vi "getAttribute_action.vi"(0 "HGF_ImaqDx":refnum<class "HGF_ImaqDx.lvclass">, 1 "Attribute Name":string, 5 "error in (no error)":errorcluster) -> (14 "dup HGF_ImaqDx":refnum<class "HGF_ImaqDx.lvclass">, 15 "IMAQdx Attribute":variant, 19 "error out":errorcluster)   [LabVIEW 2014, in "HGF_IMAQ.lvlib" / "HGF_ImaqDx.lvclass"]
doc: "Return the name of camera."
uses:
  HGF_ImaqDx.lvclass
  HGF_IMAQDevice/HGF_IMAQDevice.lvclass
  HGF_Auxiliary/HGF_Auxiliary.lvlib
  HGF_Auxiliary/Severity.ctl
  HGF_Auxiliary/ErrorCode.ctl
  VisionTools/HGF_VisionTools/HGF_VisionTools.lvlib
  VisionTools/HGF_VisionTools/IMAQdx_getAttribute_Bool.vi
  VisionTools/HGF_VisionTools/IMAQdx_getAttribute_I64.vi
  VisionTools/HGF_VisionTools/IMAQdx_getAttribute_Dbl.vi
  VisionTools/HGF_VisionTools/IMAQdx_getAttribute_U32.vi
  VisionTools/HGF_VisionTools/IMAQdx_getAttribute_Str.vi
  VisionTools/HGF_VisionTools/IMAQdx_getAttribute_Enum.vi
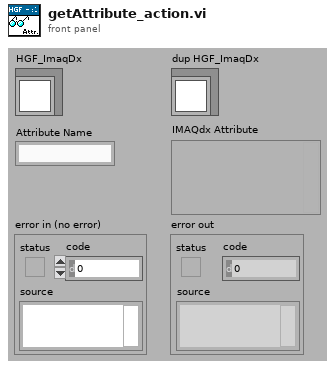
[diagram p1: front panel]
types:
  T1 = typedef "HGF_Auxiliary.lvlib/ErrorCode.ctl" = enum32{"No error", "Function not supported.", "This VI is for friends only.", "Reference object aready exisits.", "Parameter out of range.", "Not a rendezvous.", "Invalid notifier reference.", "Invalid queue reference.", "Self-Test not supported.", "Reset not supported.", "IDN query not supported.", "Error query not supported.", "Incorrect addressee.", "Object already exists.", "No class name specified", "Driver not supported", "Attribute is not writable"}
  T2 = typedef "HGF_Auxiliary.lvlib/Severity.ctl" = enum16{"Info", "Warning", "Fault", "Error", "Fatal"}
  T3 = typedef "NI_Vision_Acquisition_Software.lvlib/IMAQdx Attribute Type.ctl" = enum32{"U32", "I64", "DBL", "String", "Enum", "Bool", "Command"}
  T4 = cluster{"Attribute Type":T3, "Readable":bool, "Writable":bool, "Attribute Name":string}[]
  T5 = cluster{"Attribute Type":T3, "Readable":bool, "Writable":bool, "Attribute Name":string}
  T6 = typedef "IMAQdx.ctl" = refnum<k21>
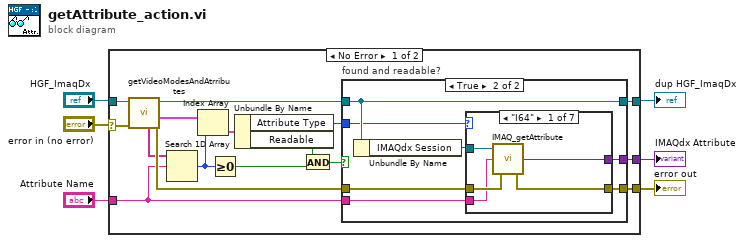
[diagram p0: block diagram]
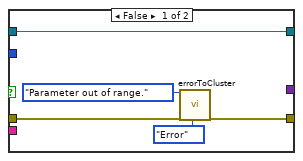
[diagram p2: hidden frame]
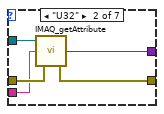
[diagram p3: hidden frame]
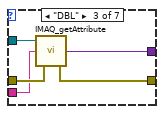
[diagram p4: hidden frame]
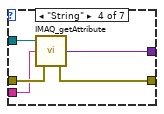
[diagram p5: hidden frame]
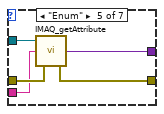
[diagram p6: hidden frame]
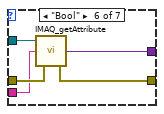
[diagram p7: hidden frame]
diagram:
  n1 = case shown="No Error" "error in (no error)" {
    selector: "error in (no error)" -> [w11 w66]
    tunnel: "HGF_ImaqDx" -> [w22 w67]
    tunnel: [w9 w67] -> w5
    tunnel: [w20 w66] -> w4
    tunnel: "Attribute Name" -> [w17 _]
    tunnel: [w7 _] -> w1
    frame No Error {
      n2 = call "getVideoModesAndAtrributes.vi"("error in (no error)"=w11, "HGF_IMAQDevice in"=w22) -> ("error out"=w19:errorcluster, "Attribute Information"=w16:T4, "HGF_IMAQDevice out"=w21:refnum<class "HGF_ImaqDx.lvclass">, "Attribute Names"=w18:string[])  [unwired: 5 in, 1 out]
      n3 = Search 1D Array(1D array=w18, element=w17) -> (index of element=w13:i32)  [unwired: 1 in]
      n4 = Index Array(array=w16, index=w13) -> (element=w15:T5)
      n5 = Greater Or Equal To 0?(x=w13) -> (x >= 0?=w12:bool)
      n6 = Unbundle By Name(w15) -> ("Attribute Type"=w8:T3, "Readable"=w14:bool)
      n7 = And(x=w14, y=w12) -> (x .and. y?=w10:bool)
      n8 = case "found and readable?" shown="True" w10 {
        tunnel: w21 -> [w27 w34]
        tunnel: [w23 w31] -> w20
        tunnel: w19 -> [w24 w32]
        tunnel: w17 -> [_ w30]
        tunnel: [w27 w34] -> w9
        tunnel: w8 -> [_ w29]
        tunnel: [_ w28] -> w7
        frame False {
          n9 = call "errorToCluster.vi"("error code"=ErrorCode."Parameter out of range.", "error in (no error)"=w24, "severity (Error)"=Severity."Error") -> ("error out"=w23:errorcluster)  [unwired: 2 in, 14 out]
        }
        frame True {
          n10 = Unbundle By Name(w34) -> ("IMAQdx Session"=w33:T6)
          n11 = case shown="\"I64\"" w29 {
            tunnel: w33 -> [w39 w44 w49 w54 w59 w64 _]
            tunnel: w32 -> [w38 w43 w48 w53 w58 w63 w65]
            tunnel: [w37 w42 w47 w52 w57 w62 w65] -> w31
            tunnel: w30 -> [w36 w41 w46 w51 w56 w61 _]
            tunnel: [w35 w40 w45 w50 w55 w60 _] -> w28
            frame "I64" {
              n12 = call-poly "IMAQ_getAttribute.vi"("error in (no error)"=w38, "Attribute Name"=w36, "IMAQdx Session"=w39) -> ("error out"=w37:errorcluster, "IMAQdx Attribute"=w35:variant)  [unwired: 1 out]
            }
            frame "U32" {
              n13 = call-poly "IMAQ_getAttribute.vi"("error in (no error)"=w43, "Attribute Name"=w41, "IMAQdx Session"=w44) -> ("error out"=w42:errorcluster, "IMAQdx Attribute"=w40:variant)  [unwired: 1 out]
            }
            frame "DBL" {
              n14 = call-poly "IMAQ_getAttribute.vi"("error in (no error)"=w48, "Attribute Name"=w46, "IMAQdx Session"=w49) -> ("error out"=w47:errorcluster, "IMAQdx Attribute"=w45:variant)  [unwired: 1 out]
            }
            frame "String" {
              n15 = call-poly "IMAQ_getAttribute.vi"("error in (no error)"=w53, "Attribute Name"=w51, "IMAQdx Session"=w54) -> ("error out"=w52:errorcluster, "IMAQdx Attribute"=w50:variant)  [unwired: 1 out]
            }
            frame "Enum" {
              n16 = call-poly "IMAQ_getAttribute.vi"("error in (no error)"=w58, "Attribute Name"=w56, "IMAQdx Session"=w59) -> ("error out"=w57:errorcluster, "IMAQdx Attribute"=w55:variant)  [unwired: 1 out]
            }
            frame "Bool" {
              n17 = call-poly "IMAQ_getAttribute.vi"("error in (no error)"=w63, "Attribute Name"=w61, "IMAQdx Session"=w64) -> ("error out"=w62:errorcluster, "IMAQdx Attribute"=w60:variant)  [unwired: 1 out]
            }
            frame "Command", Default {
            }
          }
        }
      }
    }
    frame Error {
    }
  }
  "error out" <- w4
  "dup HGF_ImaqDx" <- w5
  "IMAQdx Attribute" <- w1
